vi "DeQue.vi"(8 "ErrorArray":errorcluster[](array[cluster])) -> (0 "ErrorArray":errorcluster[](array[cluster]), 1 "Data":variant, 2 "Message":string)   [LabVIEW 2014, in "Test.lvclass"]
uses:
  Test.lvclass
  clQueMsgType.ctl
  <vilib>/Utility/error.llb/Error Cluster From Error Code.vi
  <vilib>/ErrorRing/Error Ring.xnode
  <userlib>/NIST/NISTErrorLib/NISTErrorLib.lvlib
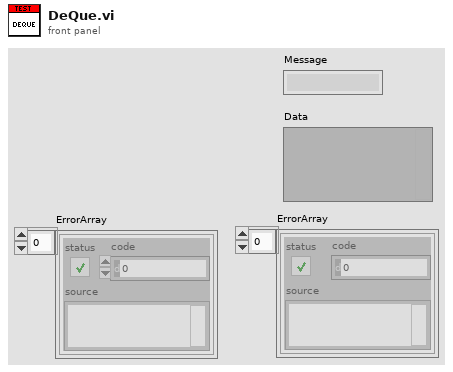
[diagram p1: front panel]
types:
  T1 = typedef "Test.lvclass/clQueMsgType.ctl" = cluster{"Message":string, "Data":variant}
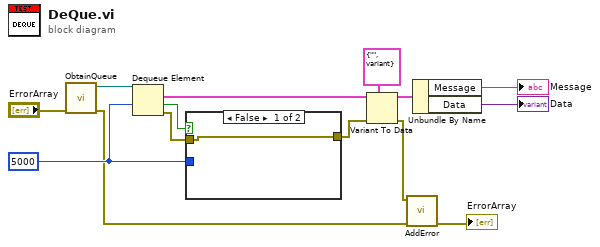
[diagram p0: block diagram]
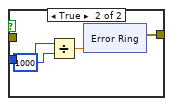
[diagram p2: hidden frame]
diagram:
  w11 = 5000 ("timeout in ms (-1)")
  n1 = call "ObtainQueue.vi"("ErrorArray"="ErrorArray") -> ("ErrorArray."=w6:errorcluster[], "TstQue"=w13:refnum<queue>)  [unwired: 9 in]
  n2 = Dequeue Element(queue=w13, timeout in ms (-1)=w11) -> (element=w8:T1, timed out?=w12:bool, error out=w10:errorcluster)  [unwired: 1 in, 1 out]
  n3 = case shown="False" w12 {
    tunnel: w11 -> [_ w19]
    tunnel: [w15 w16] -> w7
    tunnel: w10 -> [w15 _]
    frame False {
    }
    frame True {
      n4 = Divide(x=w19, y=1000) -> (x/y=w17:dbl)
      n5 = xnode "Error Ring"("parameter 0"=w17) -> ("error out"=w16:errorcluster)
    }
  }
  n6 = Variant To Data(error in=w7, type=T1 {"Message"="", "Data"=variant} ("clQueMsgType"), Variant=w8) -> (data=w3:T1, error out=w5:errorcluster)
  n7 = call <userlib>:"AddError.vi"("ErrorArray"=w6, "error in (no error)"=w5) -> ("ErrorArray"=→"ErrorArray":errorcluster[])  [unwired: 8 in, 1 out]
  n8 = Unbundle By Name(w3) -> ("Message"=→"Message":string, "Data"=→"Data":variant)
